vi "test_Remove Static Scalar Input Channels.vi"(8 "error in (no error)":errorcluster, 11 "TestCase in":refnum<class "FPGA Addon Adding Channel Items Unit Tests.lvclass">) -> (0 "error out":errorcluster, 3 "TestCase out":refnum<class "FPGA Addon Adding Channel Items Unit Tests.lvclass">)   [LabVIEW 2018, in "FPGA Addon Adding Channel Items Unit Tests.lvclass"]
uses:
  FPGA Addon Adding Channel Items Unit Tests.lvclass
  Addon/Addon System Explorer/Types/SE UI Cluster.ctl
  <vilib>/NI Veristand/Custom Device API/Custom Device Item Ref.ctl
  FPGA Addon Adding Channel Items Unit Tests.lvclass/FPGA Addon Adding Channel Items Unit Tests.ctl
  Addon/Addon Shared/SubVIs/Constants.vi
  <vilib>/NI Veristand/Custom Device Tools/Custom Device Utility Library/NI VeriStand - Search for Item by GUID.vi
  <vilib>/NI/NI VeriStand Advanced SysDef API/_SubVIs/SysDef.Search.GUIDs.vi
  <vilib>/addons/_JKI Toolkits/VI Tester/TestCase.llb/TestCase.lvclass
  <vilib>/NI Veristand/Custom Device Tools/Custom Device Utility Library/Custom Device Utility Library.lvlib
  Addon/Addon Shared/FPGA Addon Shared.lvlib
  <vilib>/NI/NI VeriStand Advanced SysDef API/SysDef API/Advanced System Definition.lvlib
  Addon/Addon System Explorer/FPGA Addon System Explorer.lvlib
  <vilib>/NI Veristand/Custom Device API/Custom Device API.lvlib
  C:/Program Files (x86)/National Instruments/LabVIEW 2018/vi.lib/addons/_JKI Toolkits/VI Tester/TestCase.llb/TestCase.lvclass
panel:
  out "GUIDs":string[](array[string])
  in  "remove":bool
  in  "add":bool
  out "Names":string[](array[string])
  in  "Available Registers":i32[](listbox)
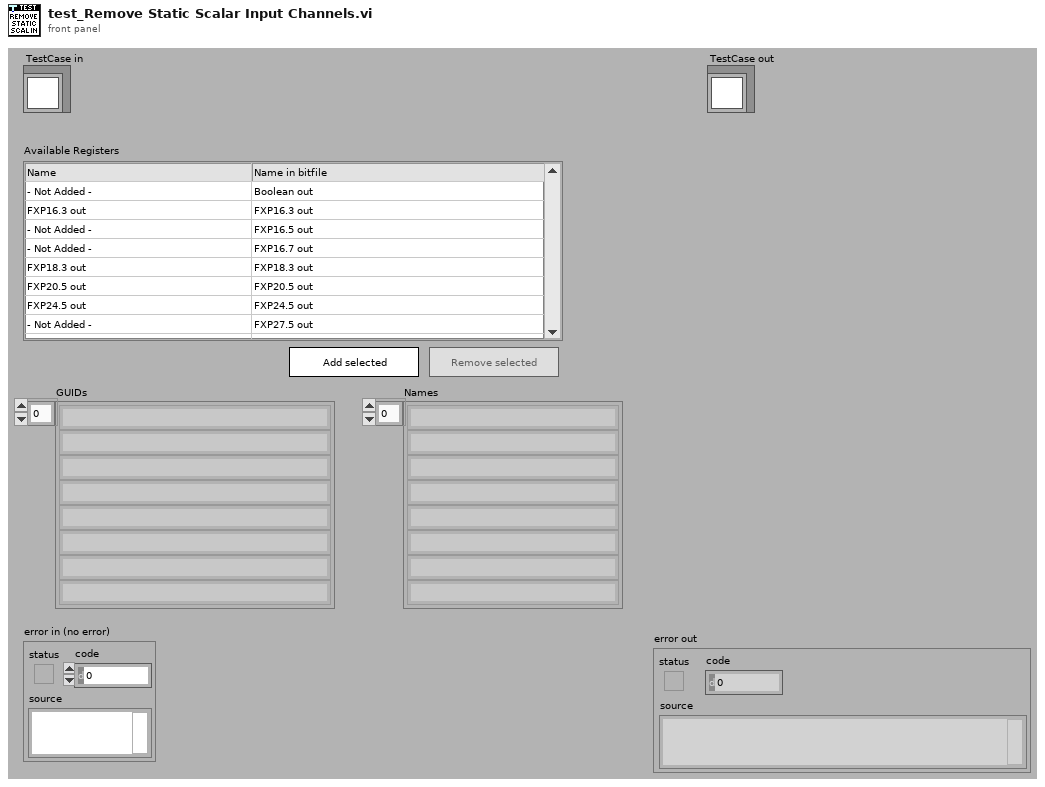
[diagram p1: front panel]
types:
  T1 = typedef "FPGA Addon System Explorer.lvlib/SE UI Cluster.ctl" = cluster{"Node Ptr":T2, "Add":refnum<vi>, "Remove":refnum<vi>, "Registers ListBox":refnum<vi>}
  T2 = typedef "Custom Device API.lvlib/Custom Device Item Ref.ctl" = u64
  T3 = typedef "Advanced System Definition.lvlib/TreeItem.Info.ctl" = cluster{"Name":string, "Description":string, "GUID":string, "Is Channel":bool, "Channel":T4, "Is Waveform":bool, "Waveform":T6}
  T4 = typedef "Custom Device API.lvlib/Custom Device Channel.ctl" = cluster{"Type":T5, "Units":string, "Default Value":dbl, "Faultable":bool, "Scalable":bool}
  T5 = typedef "Custom Device API.lvlib/Custom Device Channel Type.ctl" = enum16{"Input", "Output"}
  T6 = typedef "Custom Device API.lvlib/Custom Device Waveform.ctl" = cluster{"Data Type":T7, "Units":string}
  T7 = typedef "Custom Device API.lvlib/Custom Device Waveform DataType.ctl" = enum16{"Double", "Complex Double"}
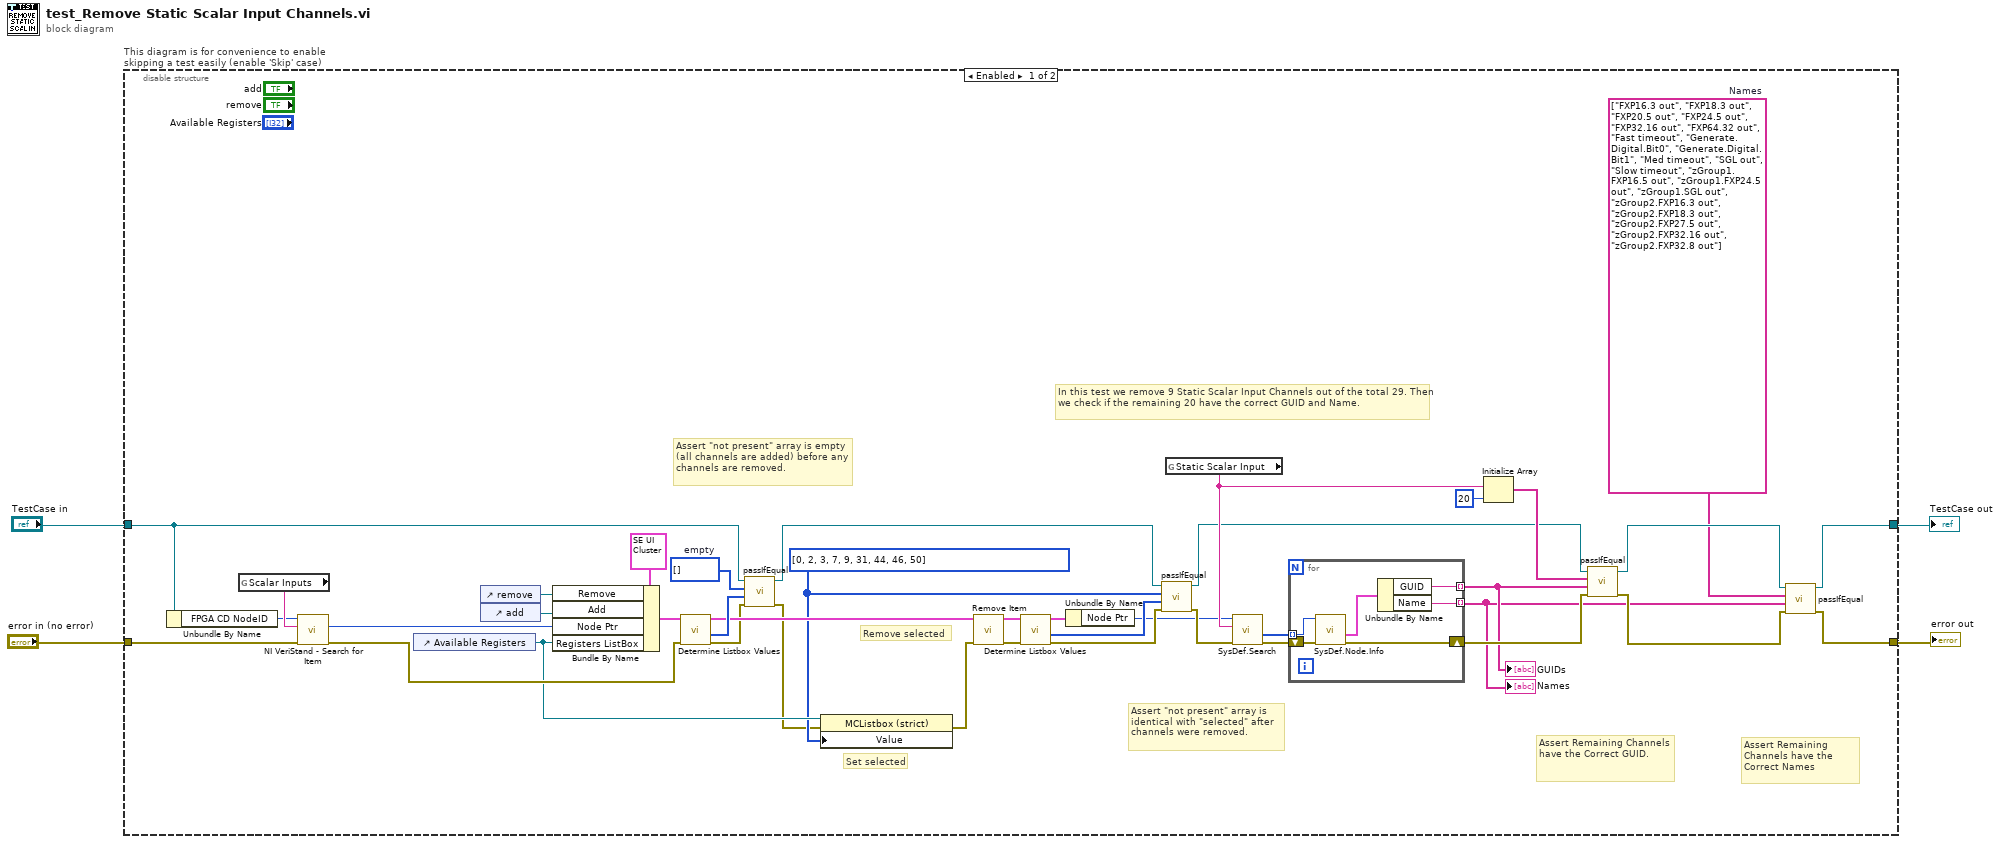
[diagram p0: block diagram]
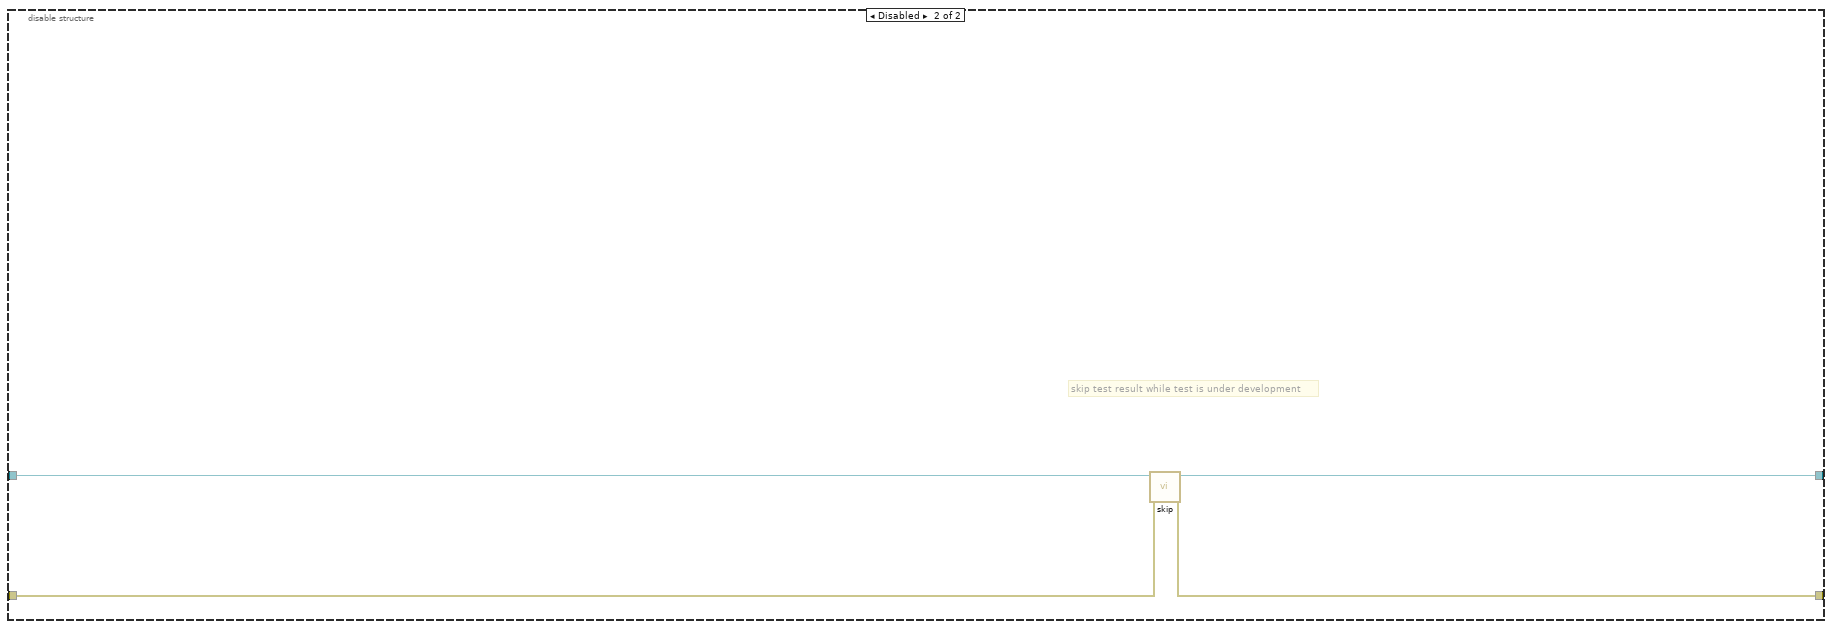
[diagram p2: hidden frame]
diagram:
  n1 = disable-structure "This diagram is for convenience to enable skipping a test easily (enable 'Skip' case)" shown="Enabled" {
    disable-tunnel: "TestCase in" -> [w25 w54]
    disable-tunnel: [w35 w52] -> w1
    disable-tunnel: [w34 w53] -> w3
    disable-tunnel: "error in (no error)" -> [w33 w51]
    frame Enabled {
      w26 = i32[] []  # empty
      w36 = string[] ["FXP16.3 out", "FXP18.3 out", "FXP20.5 out", "FXP24.5 out", "FXP32.16 out", "FXP64.32 out", "Fast timeout", "Generate.Digital.Bit0", "Generate.Digital.Bit1", "Med timeout", "SGL out", "Slow timeout", "zGroup1.FXP16.5 out", "zGroup1.FXP24.5 out", "zGroup1.SGL out", "zGroup2.FXP16.3 out", "zGroup2.FXP18.3 out", "zGroup2.FXP27.5 out", "zGroup2.FXP32.16 out", "zGroup2.FXP32.8 out"]  # Names
      w14 = i32[] [0, 2, 3, 7, 9, 31, 44, 46, 50] ("selected")
      # "Remove selected"
      # "Set selected"
      # "Assert \"not present\" array is empty (all channels are added) before any channels are removed."
      # "Assert \"not present\" array is identical with \"selected\" after channels were removed."
      # "In this test we remove 9 Static Scalar Input Channels out of the total 29. Then we check if the remaining 20 have the correct GUID and Name."
      # "Assert Remaining Channels have the Correct Names"
      # "Assert Remaining Channels have the Correct GUID."
      n2 = Unbundle By Name(w25) -> ("FPGA CD NodeID"=w32:u64)
      n3 = global read "Constants.vi" "Scalar Inputs"() -> (w44:string)
      n4 = call-poly <vilib>:"NI VeriStand - Search for Item.vi"("error in"=w33, "Item GUID"=w44, "Section Ref in"=w32) -> ("error out"=w17:errorcluster, "Item Ref"=w22:T2)  [unwired: 5 in, 2 out]
      n5 = control-ref of="Available Registers"() -> (w15:refnum<vi>)
      n6 = control-ref of="remove"() -> (w21:refnum<vi>)
      n7 = control-ref of="add"() -> (w20:refnum<vi>)
      n8 = Bundle By Name(cluster=T1 {"Node Ptr"=18446744073709551615, "Add"=refnum, "Remove"=refnum, "Registers ListBox"=refnum} ("SE UI cluster in"), "Remove"=w21, "Add"=w20, "Node Ptr"=w22, "Registers ListBox"=w15) -> (w19:T1)
      n9 = call "Determine Listbox Values.vi"("error in (no error)"=w17, "SE UI cluster in"=w19) -> ("error out"=w13:errorcluster, "Not imported item Indexes"=w18:i32[], "SE UI cluster out"=w16:T1)  [unwired: 6 in, 1 out]
      n10 = call-dynamic "passIfEqual.vi"("error in (no error)"=w13, "y"=w18, "x"=w26, "TestCase in"=w25) -> ("error out"=w12:errorcluster, "TestCase out"=w24:refnum<class "FPGA Addon Adding Channel Items Unit Tests.lvclass">)  [unwired: 6 in]
      n11 = property class="MCListbox (strict)"(reference=w15, error in=w12, "Value"=w14) -> (error out=w11:errorcluster)  [unwired: 1 out]
      n12 = call "Remove Item.vi"("error in (no error)"=w11, "SE UI cluster in"=w16) -> ("error out"=w10:errorcluster, "SE UI cluster out"=w9:T1)  [unwired: 7 in, 1 out]
      n13 = call "Determine Listbox Values.vi"("error in (no error)"=w10, "SE UI cluster in"=w9) -> ("error out"=w7:errorcluster, "Not imported item Indexes"=w8:i32[], "SE UI cluster out"=w6:T1)  [unwired: 6 in, 1 out]
      n14 = Unbundle By Name(w6) -> ("Node Ptr"=w5:T2)
      n15 = call-dynamic "passIfEqual.vi"("error in (no error)"=w7, "y"=w8, "x"=w14, "TestCase in"=w24) -> ("error out"=w28:errorcluster, "TestCase out"=w27:refnum<class "FPGA Addon Adding Channel Items Unit Tests.lvclass">)  [unwired: 6 in]
      n16 = global read "Constants.vi" "Static Scalar Input"() -> (w30:string)
      n17 = call-poly <vilib>:"SysDef.Search.vi"("error in (no error)"=w28, "GUID"=w30, "nodeID"=w5) -> ("error out"=w43:errorcluster, "Values Out"=w42:u64[])  [unwired: 5 in, 2 out]
      n18 = for {
        tunnel: w42 -> [w47] mode=indexing
        tunnel: [w45] -> w37 mode=indexing
        tunnel: [w46] -> w39 mode=indexing
        shift-right: [w49] -> w40
        shift-left: w43 -> [w50]
        n19 = call <vilib>:"SysDef.Node.Info.vi"("error in (no error)"=w50, "nodeID"=w47) -> ("error out"=w49:errorcluster, "Item Info"=w48:T3)  [unwired: 6 in, 2 out]
        n20 = Unbundle By Name(w48) -> ("GUID"=w46:string, "Name"=w45:string)
      }
      "Names" <- w37
      "GUIDs" <- w39
      n21 = Initialize Array(w30, 20 ("dimension size")) -> (w31:string[])
      n22 = call-dynamic "passIfEqual.vi"("error in (no error)"=w40, "y"=w39, "x"=w31, "TestCase in"=w27) -> ("error out"=w41:errorcluster, "TestCase out"=w38:refnum<class "FPGA Addon Adding Channel Items Unit Tests.lvclass">)  [unwired: 6 in]
      n23 = call-dynamic "passIfEqual.vi"("error in (no error)"=w41, "y"=w37, "x"=w36, "TestCase in"=w38) -> ("error out"=w34:errorcluster, "TestCase out"=w35:refnum<class "FPGA Addon Adding Channel Items Unit Tests.lvclass">)  [unwired: 6 in]
    }
    frame Disabled {
      # "skip test result while test is under development"
      n24 = call <vilib>:"skip.vi"("error in (no error)"=w51, "TestCase in"=w54) -> ("error out"=w53:errorcluster, "TestCase out"=w52:refnum<class "FPGA Addon Adding Channel Items Unit Tests.lvclass">)  [unwired: 8 in]
    }
  }
  "error out" <- w3
  "TestCase out" <- w1
